vi "Calculate Fill Path.vi"(8 "error in (no error)":errorcluster, 9 "Curve 2":T1[](array[typedef]), 10 "Curve 1":T1[](array[typedef]), 11 "Tool Funnel in":refnum<class "Tool Funnel.lvclass">) -> (0 "error out":errorcluster, 2 "Points":T1[](array[typedef]), 3 "Tool Funnel out":refnum<class "Tool Funnel.lvclass">)   [LabVIEW 2019, in "Tool Funnel.lvclass"]
uses:
  Tool Funnel.lvclass
  Parse/PathCommands/Point.ctl
  Settings/Funnel Settings/Funnel Settings.lvclass/Funnel Settings.ctl
  Settings/Funnel Settings/Funnel Settings.lvclass
  Parse/PathCommands/PathCommands.lvclass
panel:
  out "XY Graph 2":cluster{"X":dbl, "Y":dbl}[](graph)
  out "XY Graph 4":cluster{"X":dbl, "Y":dbl}[](graph)
  out "XY Graph 3":cluster{"X":dbl, "Y":dbl}[](graph)
  out "XY Graph":cluster{"X":dbl, "Y":dbl}[](graph)
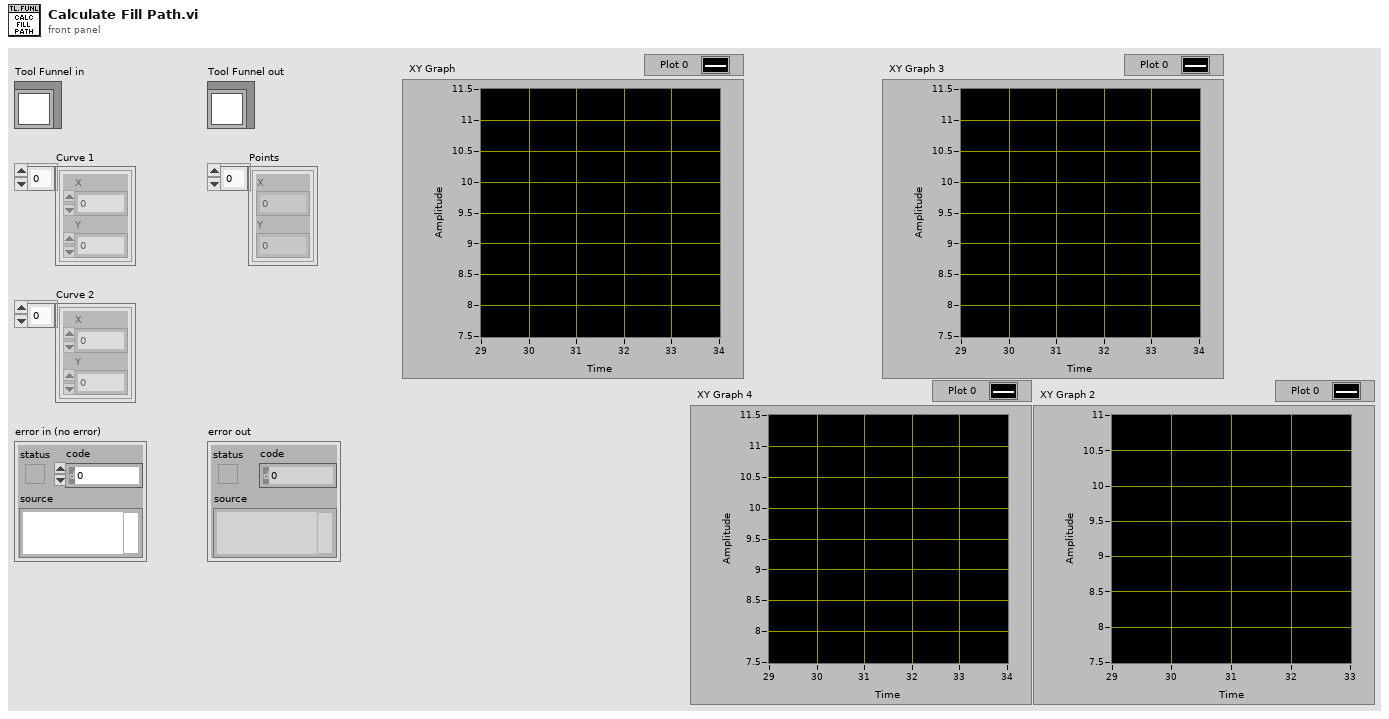
[diagram p1: front panel]
types:
  T1 = typedef "PathCommands.lvclass/Point.ctl" = cluster{"X":dbl, "Y":dbl}
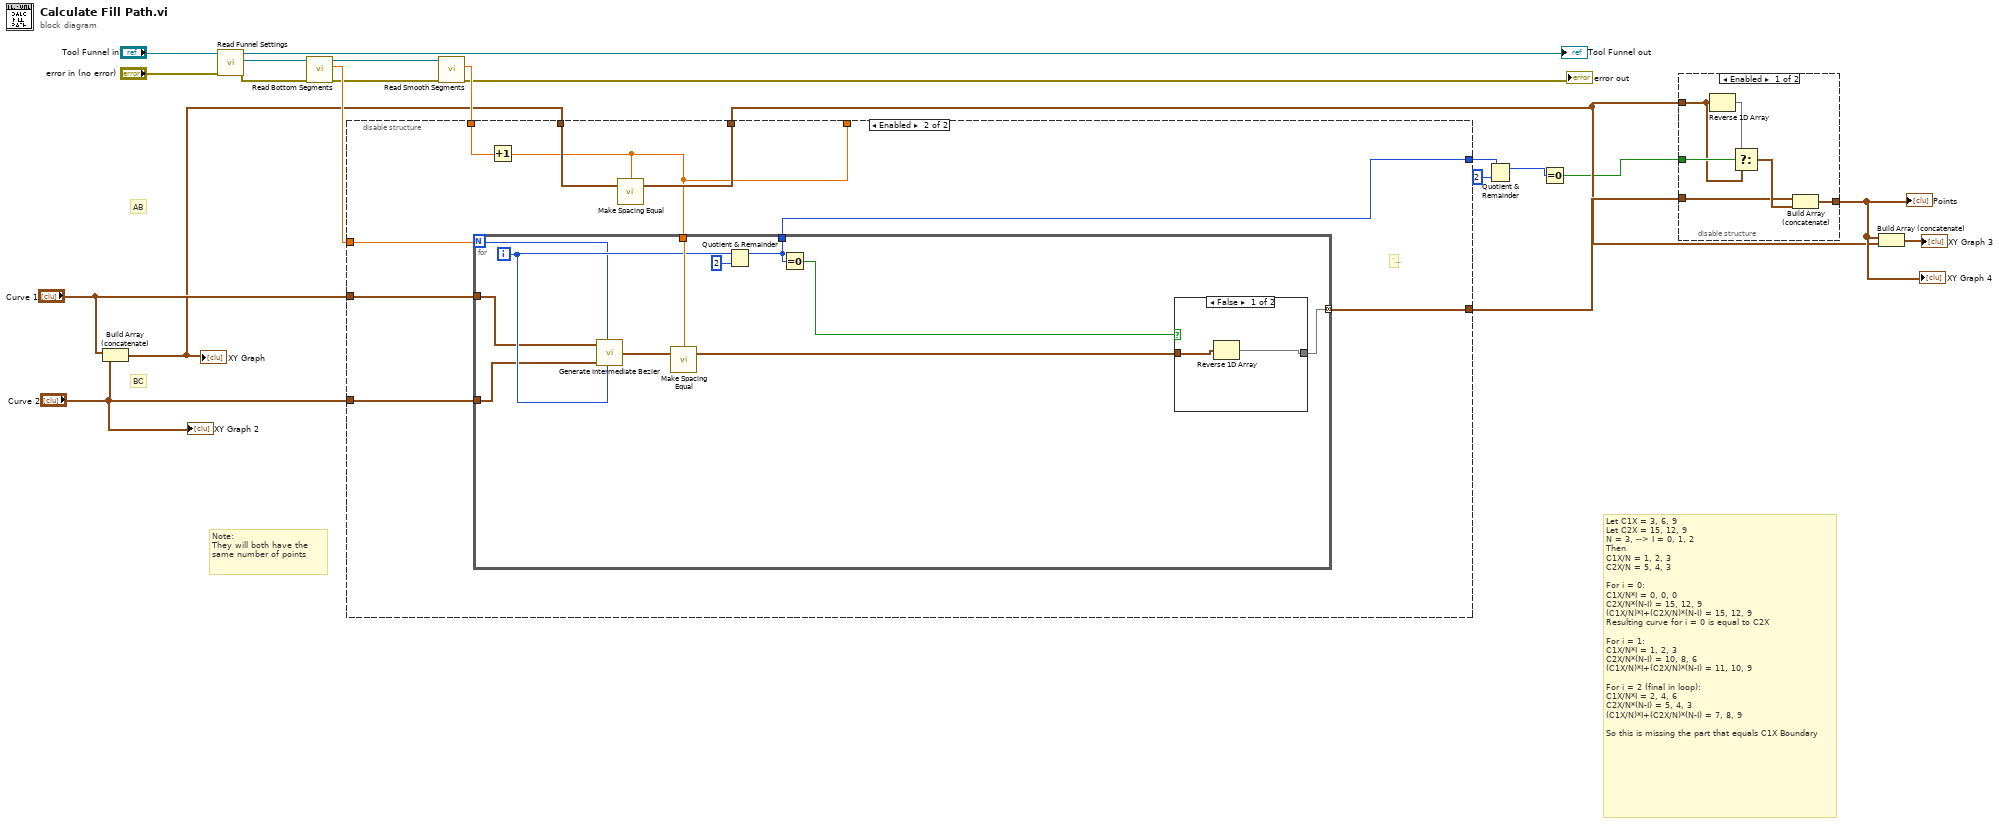
[diagram p0: block diagram]
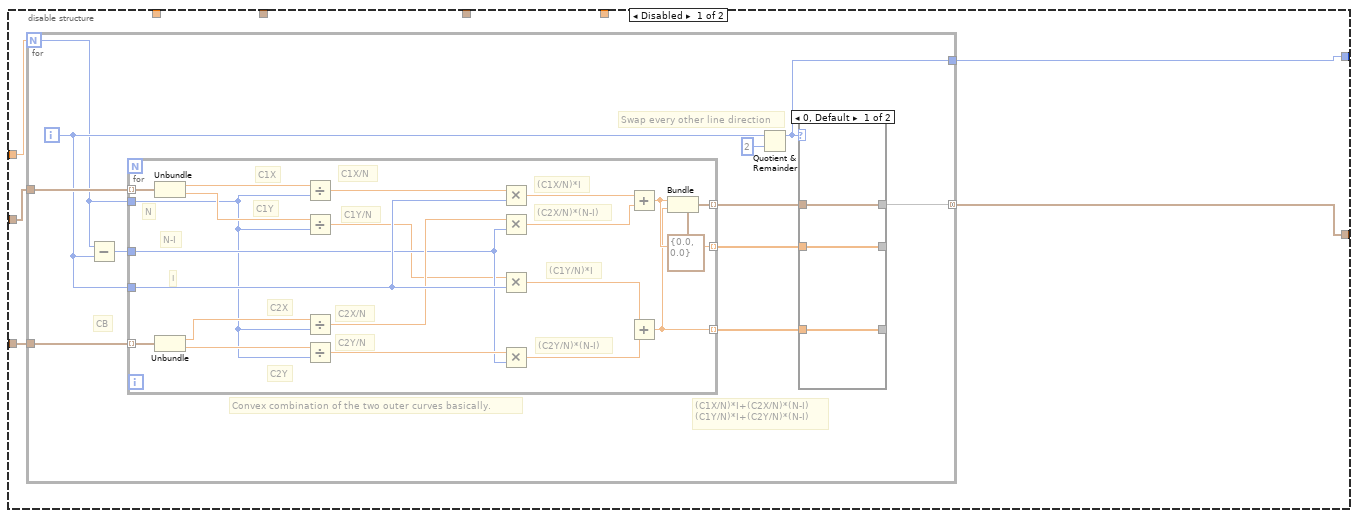
[diagram p3: hidden frame]
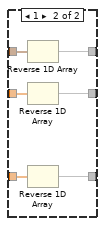
[diagram p4: hidden frame]
diagram:
  # "BC"
  # "AB"
  # "Let C1X = 3, 6, 9\nLet C2X = 15, 12, 9\nN = 3, --> I = 0, 1, 2\nThen \nC1X/N = 1, 2, 3\nC2X/N = 5, 4, 3\n\nFor i = 0:\nC1X/N*I = 0, 0, 0\nC2X/N*(N-I) = 15, 12, 9\n(C1X/N)*I+(C2X/N)*(N-I) = 15, 12, 9\nResulting curve for i = 0 is equal to C2X\n\nFor i = 1:\nC1X/N*I = 1, 2, 3\nC2X/N*(N-I) = 10, 8, 6\n(C1X/N)*I+(C2X/N)*(N-I) = 11, 10, 9\n\nFor i = 2 (final in loop):\nC1X/N*I = 2, 4, 6\nC2X/N*(N-I) = 5, 4, 3\n(C1X/N)*I+(C2X/N)*(N-I) = 7, 8, 9\n\nSo this is missing the part that equals C1X Boundary"
  # "Note:\nThey will both have the same number of points"
  n1 = Build Array (concatenate)("Curve 1", "Curve 2") -> (w6:T1[])
  "XY Graph" <- w6
  n2 = call-dynamic "Read Funnel Settings.vi"("error in (no error)"="error in (no error)", "Tool Funnel in"="Tool Funnel in") -> ("error out"=w17:errorcluster, "Funnel Settings.lvclass"=w19:refnum<class "Funnel Settings.lvclass">, "Tool Funnel out"=→"Tool Funnel out":refnum<class "Tool Funnel.lvclass">)  [unwired: 7 in]
  n3 = call "Read Bottom Segments.vi"("error in (no error)"=w17, "Funnel Settings in"=w19) -> ("error out"=w13:errorcluster, "Bottom Segments"=w18:dbl, "Funnel Settings out"=w12:refnum<class "Funnel Settings.lvclass">)  [unwired: 7 in]
  n4 = call "Read Smooth Segments.vi"("error in (no error)"=w13, "Funnel Settings in"=w12) -> ("error out"=→"error out":errorcluster, "Smooth Segments"=w14:dbl)  [unwired: 7 in, 1 out]
  n5 = disable-structure shown="Enabled" {
    disable-tunnel: [w26 w73] -> w3
    disable-tunnel: w18 -> [w25 w71]
    disable-tunnel: "Curve 2" -> [w24 w75]
    disable-tunnel: [w23 w74] -> w15
    disable-tunnel: "Curve 1" -> [w22 w76]
    disable-tunnel: [_ w68] -> _
    disable-tunnel: w14 -> [_ w72]
    disable-tunnel: w6 -> [_ w70]
    disable-tunnel: [_ w69] -> w5
    frame Disabled {
      n6 = for {
        N: w25 -> [w31]
        tunnel: w24 -> [w30]
        tunnel: w22 -> [w35]
        tunnel: [w32] -> w26
        tunnel: [w29] -> w23 mode=concatenating
        i -> [w34]
        # "Convex combination of the two outer curves basically."
        # "CB"
        # "Swap every other line direction"
        # "(C1X/N)*I+(C2X/N)*(N-I)\n(C1Y/N)*I+(C2Y/N)*(N-I)"
        n7 = Subtract(x=w31, y=w34) -> (x-y=w37:i32)
        n8 = for {
          tunnel: w35 -> [w67] mode=indexing
          tunnel: w30 -> [w66] mode=indexing
          tunnel: w34 -> [w62]
          tunnel: w37 -> [w57]
          tunnel: [w53] -> w33 mode=indexing
          tunnel: w31 -> [w52]
          tunnel: [w48] -> w28 mode=indexing
          tunnel: [w47] -> w27 mode=indexing
          # "C2Y"
          # "I"
          # "N"
          # "N-I"
          # "(C2Y/N)*(N-I)"
          # "C2Y/N"
          # "(C2X/N)*(N-I)"
          # "C2X/N"
          # "C2X"
          # "(C1Y/N)*I"
          # "C1Y/N"
          # "C1Y"
          # "(C1X/N)*I"
          # "C1X/N"
          # "C1X"
          n9 = Unbundle(w67) -> ("X"=w65:dbl, "Y"=w63:dbl)
          n10 = Unbundle(w66) -> ("X"=w61:dbl, "Y"=w60:dbl)
          n11 = Divide(x=w65, y=w52) -> (x/y=w64:dbl)
          n12 = Divide(x=w63, y=w52) -> (x/y=w51:dbl)
          n13 = Divide(x=w61, y=w52) -> (x/y=w59:dbl)
          n14 = Divide(x=w60, y=w52) -> (x/y=w58:dbl)
          n15 = Multiply(x=w64, y=w62) -> (x*y=w56:dbl)
          n16 = Multiply(x=w59, y=w57) -> (x*y=w55:dbl)
          n17 = Multiply(x=w51, y=w62) -> (x*y=w54:dbl)
          n18 = Multiply(x=w58, y=w57) -> (x*y=w50:dbl)
          n19 = Add(x=w56, y=w55) -> (x+y=w48:dbl)
          n20 = Add(x=w54, y=w50) -> (x+y=w47:dbl)
          n21 = Bundle(cluster=T1 {"X"=0.0, "Y"=0.0} ("Point"), "X"=w48, "Y"=w47) -> (w53:T1)
        }
        n22 = Quotient & Remainder(x=w34, y=2) -> (x-y*floor(x/y)=w32:i32)  [unwired: 1 out]
        n23 = case shown="0, Default" w32 {
          tunnel: w33 -> [w40 w46]
          tunnel: [w40 w45] -> w29
          tunnel: w28 -> [w39 w44]
          tunnel: w27 -> [w38 w43]
          tunnel: [w39 w42] -> _
          tunnel: [w38 w41] -> _
          frame 0, Default {
          }
          frame 1 {
            n24 = Reverse 1D Array(array=w46) -> (reversed array=w45:T1[])
            n25 = Reverse 1D Array(array=w44) -> (reversed array=w42:dbl[])
            n26 = Reverse 1D Array(array=w43) -> (reversed array=w41:dbl[])
          }
        }
      }
    }
    frame Enabled {
      # "``"
      n27 = Increment(x=w72) -> (x+1=w68:dbl)
      n28 = for {
        N: w71 -> [w77]
        tunnel: w68 -> [w83]
        tunnel: w76 -> [w78]
        tunnel: w75 -> [w79]
        tunnel: [w85] -> w74 mode=concatenating
        tunnel: [w84] -> w73
        i -> [w80]
        n29 = call "Generate Intermediate Bezier.vi"("Curve 1"=w78, "N"=w77, "Curve 2"=w79, "I"=w80) -> ("Curve I"=w81:T1[])  [unwired: 3 in]
        n30 = call "Make Spacing Equal.vi"("Points"=w81, "Smooth Points"=w83) -> ("Evenly spaced"=w82:T1[])  [unwired: 1 in]
        n31 = Quotient & Remainder(x=w80, y=2) -> (x-y*floor(x/y)=w84:i32)  [unwired: 1 out]
        n32 = Equal To 0?(x=w84) -> (x = 0?=w86:bool)
        n33 = case shown="False" w86 {
          tunnel: w82 -> [w89 w90]
          tunnel: [w88 w90] -> w85
          frame False {
            n34 = Reverse 1D Array(array=w89) -> (reversed array=w88:T1[])
          }
          frame True {
          }
        }
      }
      n35 = call "Make Spacing Equal.vi"("Points"=w70, "Smooth Points"=w68) -> ("Evenly spaced"=w69:T1[])  [unwired: 1 in]
    }
  }
  n36 = Quotient & Remainder(x=w3, y=2) -> (x-y*floor(x/y)=w1:i32)  [unwired: 1 out]
  n37 = Equal To 0?(x=w1) -> (x = 0?=w2:bool)
  n38 = disable-structure shown="Enabled" {
    disable-tunnel: w2 -> [w96 _]
    disable-tunnel: [w93 w97] -> w8
    disable-tunnel: w15 -> [w92 w97]
    disable-tunnel: w5 -> [w91 _]
    frame Enabled {
      n39 = Reverse 1D Array(array=w91) -> (reversed array=w95:T1[])
      n40 = Select(t=w95, s=w96, f=w91) -> (s? t:f=w94:T1[])
      n41 = Build Array (concatenate)(w92, w94) -> (w93:T1[])
    }
    frame Disabled {
    }
  }
  "Points" <- w8
  "XY Graph 4" <- w8
  n42 = Build Array (concatenate)(w8, w5) -> (→"XY Graph 3":T1[])
  "XY Graph 2" <- "Curve 2"
